vi "UserConsole_Main.vi"(8 "error in (no error)":errorcluster) -> (0 "error out":errorcluster)   [LabVIEW 2013]
doc: "This is Top Level VI for User Console Module. You can communicate with this module using its API. Communication is made based on queue. This module has User Interface so I chase Producer Consumer architecture. In this architecture the User Interface loop is closed using User Event. User Event is sent by Processing (Consumer) loop."
uses:
  General/Controls/#TD_General_CommunicationQueueStates_Enum.ctl
  Private controls/#TD_UserConsole_InnerData_Cluster.ctl
  Private controls/#TD_UserConsole_ModuleStates_Enum.ctl
  Private controls/#TD_UserConsole_ModuleData_Cluster.ctl
  General/Controls/#TD_General_FromWho_Enum.ctl
  General/Controls/#TD_General_UserEventStates_Enum.ctl
  Private controls/#TD_UserConsole_Transactions_Cluster.ctl
  Private controls/#TD_UserConsole_Keys_Cluster.ctl
panel:
  out "CardReader":bool
  in  "Transactions":T1
  in  "blanck_picture":cluster{"Keys":T2, "Screen":string} caption="blank_picture"
  # "[Covers: UI1]"
  # "[Covers: UI2] \n[Covers: UI2A] \n[Covers: UI2B]\n[Covers: UI2C]"
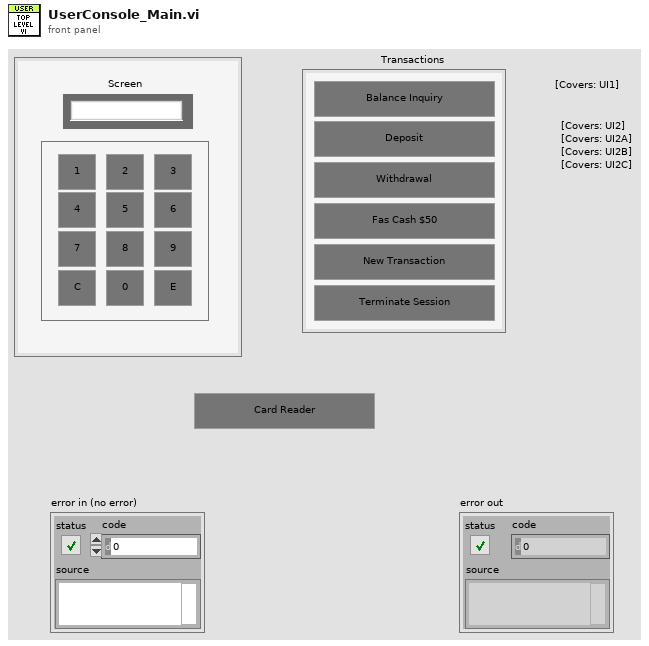
[diagram p1: front panel]
types:
  T1 = typedef "#TD_UserConsole_Transactions_Cluster.ctl" = cluster{"BalanceInquiry":bool, "Deposit":bool, "Withdrawal":bool, "FastCash50":bool, "NewTransaction":bool, "TerminateSession":bool}
  T2 = typedef "#TD_UserConsole_Keys_Cluster.ctl" = cluster{"B1":bool, "B2":bool, "B3":bool, "B4":bool, "B5":bool, "B6":bool, "B7":bool, "B8":bool, "B9":bool, "BC":bool, "B0":bool, "BE":bool}
  T3 = typedef "#TD_General_UserEventStates_Enum.ctl" = enum16{"ERROR_Default", "Create", "GetRef", "Generate", "Release"}
  T4 = typedef "#TD_General_CommunicationQueueStates_Enum.ctl" = enum16{"ERROR_Default", "Obtain", "GetRef", "Enqueue", "EnqueueAtOpp", "GetStatus", "Release"}
  T5 = typedef "#TD_General_FromWho_Enum.ctl" = enum16{"ERROR_Default", "UserConsole", "DisplayConsole", "SensorInterface", "Controller", "Database", "Timing", "ErrorHandling"}
  T6 = typedef "#TD_UserConsole_ModuleStates_Enum.ctl" = enum16{"ERROR_Default", "Init", "Close", "ErrorHandling", "KeyPressed", "TransactionPressed", "CardReaderPressed", "UpdateFP"}
  T7 = typedef "#TD_UserConsole_ModuleData_Cluster.ctl" = cluster{"Action":T6, "Data":variant}
  T8 = typedef "#TD_General_IntermoduleData_Cluster.ctl" = cluster{"Sender":T5, "ModuleData":variant}
  T9 = typedef "#TD_UserConsole_InnerData_Cluster.ctl" = cluster{"Sth":bool, "Screen":string}
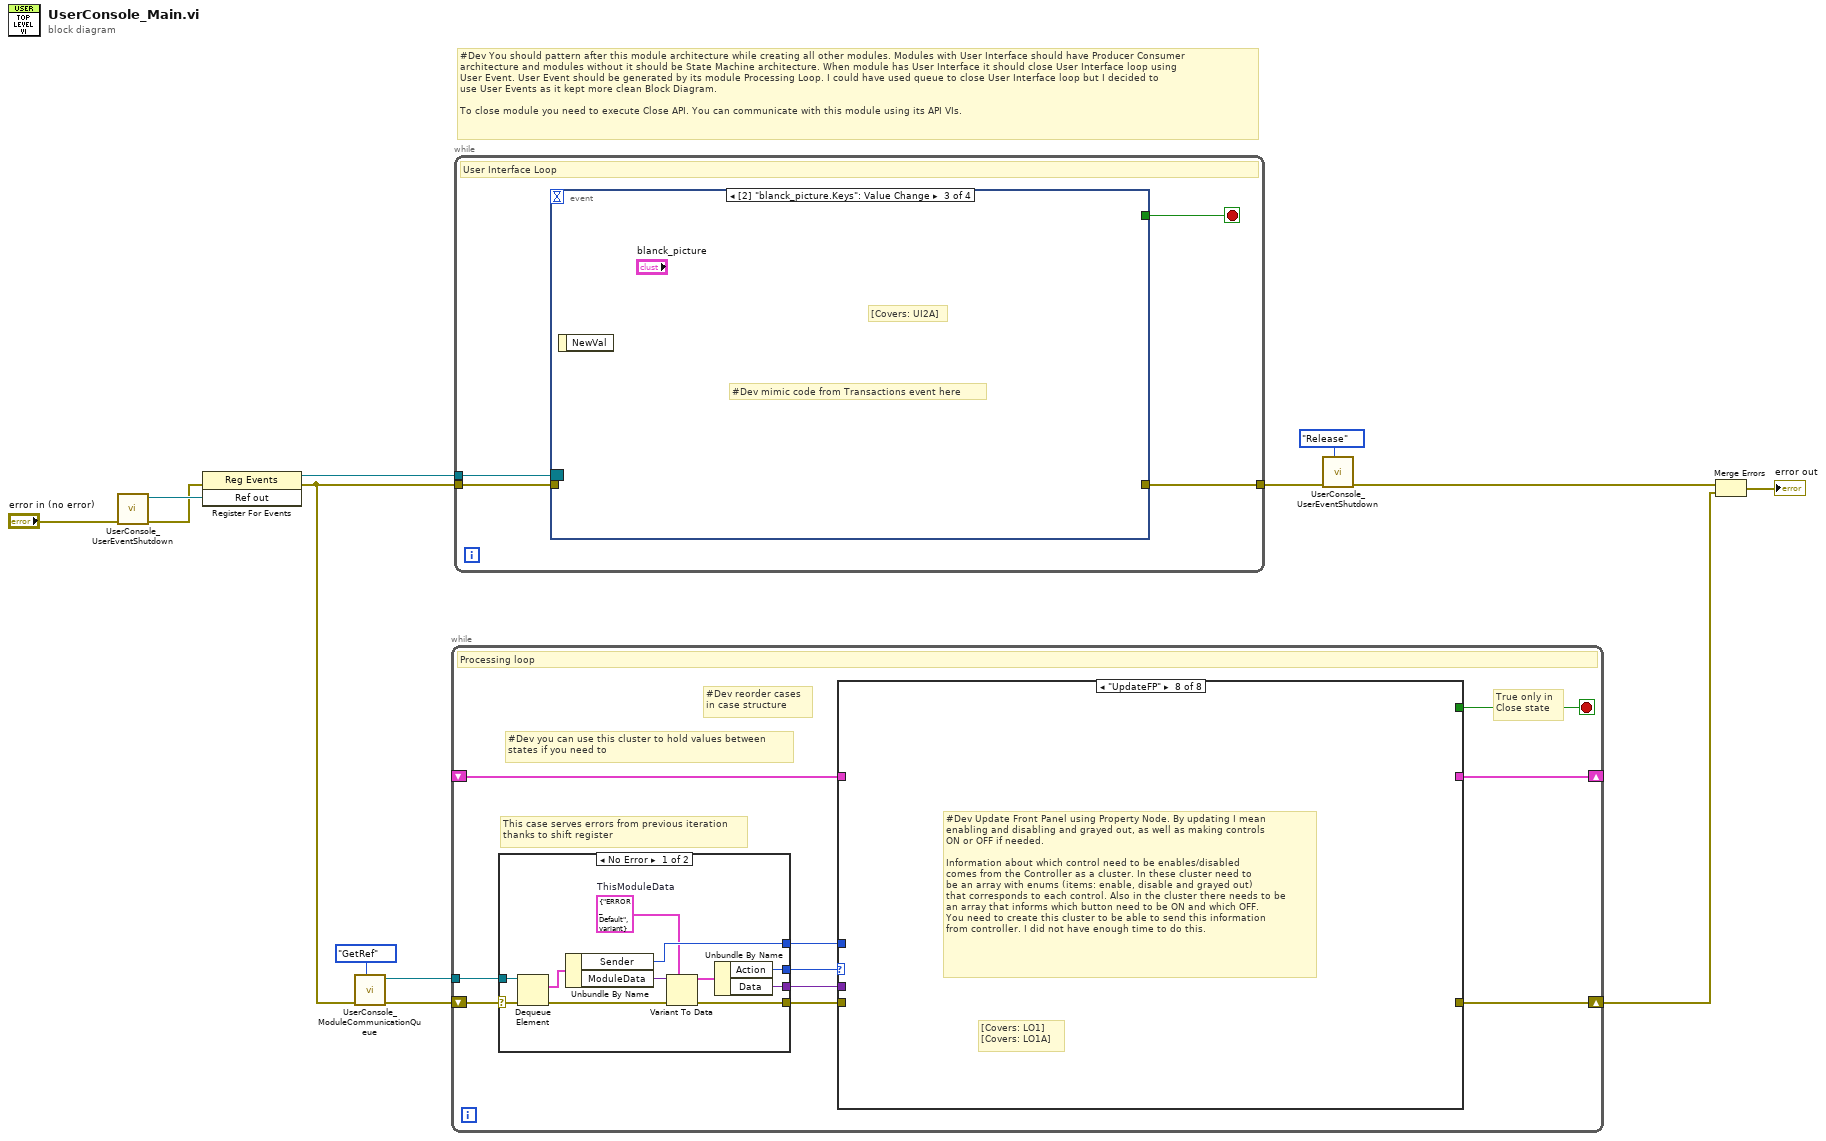
[diagram p0: block diagram]
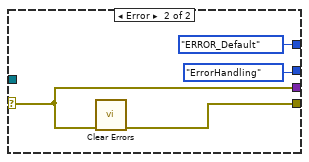
[diagram p2: hidden frame]
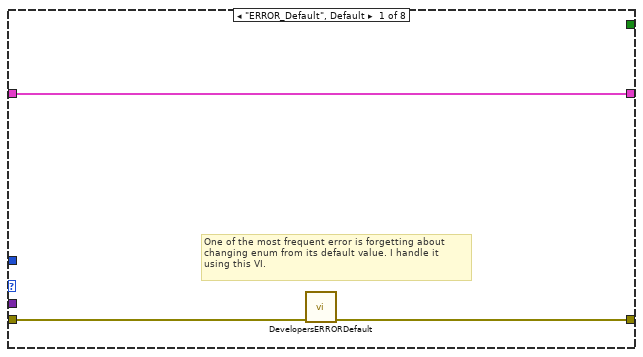
[diagram p3: hidden frame]
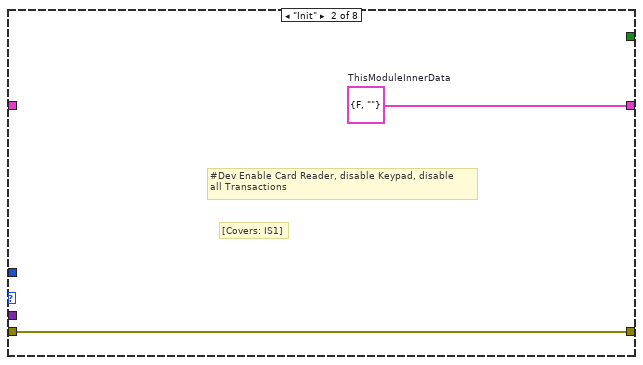
[diagram p4: hidden frame]
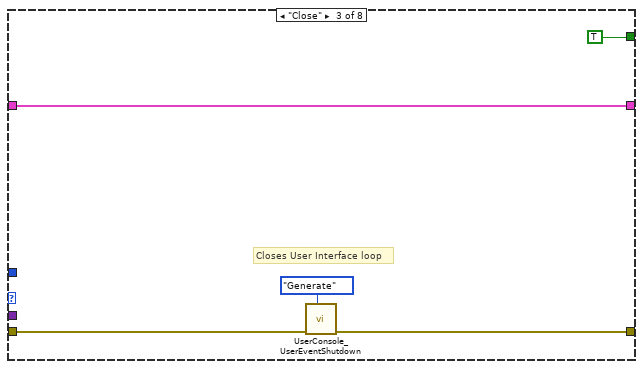
[diagram p5: hidden frame]
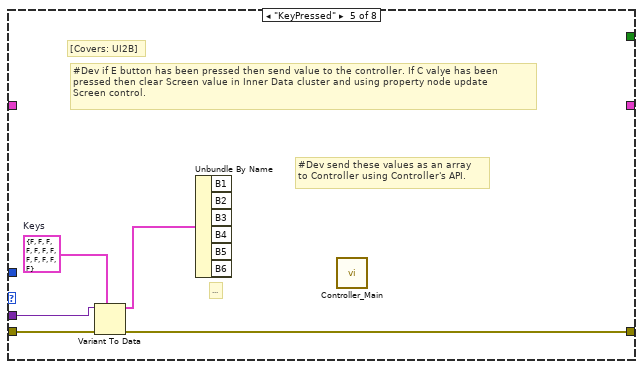
[diagram p7: hidden frame]
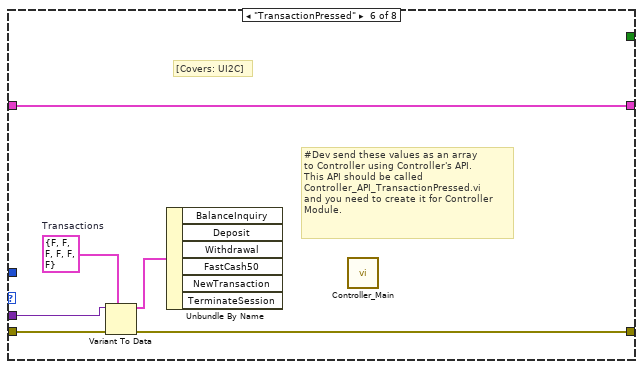
[diagram p8: hidden frame]
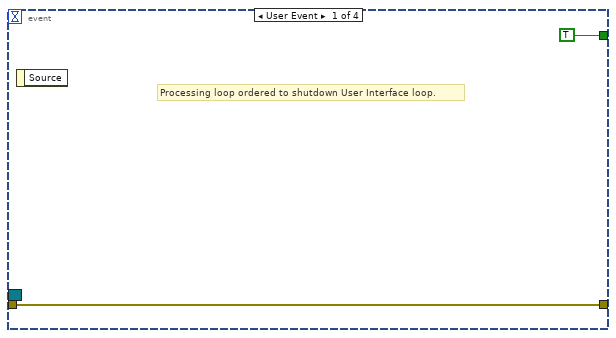
[diagram p10: hidden frame]
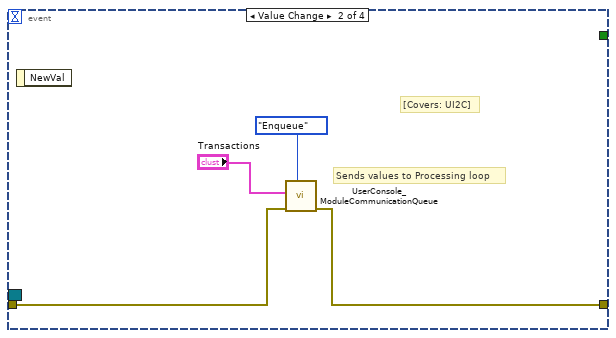
[diagram p11: hidden frame]
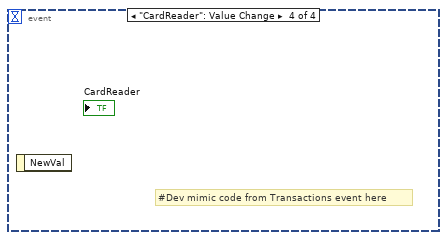
[diagram p12: hidden frame]
diagram:
  # "#Dev You should pattern after this module architecture while creating all other modules. Modules with User Interface should have Producer Consumer \narchitecture and modules without it should be State Machine architecture. When module has User Interface it should close User Interface loop using \nUser Event. User Event should be generated by its module Processing Loop. I could have used queue to close User Interface loop but I decided to \nuse User Events as it kept more clean Block Diagram.\n\nTo close module you need to execute Close API. You can communicate with this module using its API VIs."
  n1 = call "UserConsole_UserEventShutdown.vi"("error in (no error)"="error in (no error)") -> ("error out"=w12:errorcluster, "Ref out"=w13:refnum<user-event>)  [unwired: 9 in]
  n2 = register-events(error in=w12, w13) -> (reference out=w11:refnum<event-registration>, error out=w9:errorcluster)  [unwired: 1 in]
  n3 = call "UserConsole_ModuleCommunicationQueue.vi"("Action"=#TD_General_CommunicationQueueStates_Enum."GetRef", "error in (no error)"=w9) -> ("error out"=w1:errorcluster, "Ref out"=w7:refnum<queue>)  [unwired: 7 in, 1 out]
  n4 = while {
    tunnel: w7 -> [w22]
    shift-right: [w15] -> w3
    shift-left: w1 -> [w23]
    shift-right: [w21] -> _
    shift-left: _ -> [w20]
    stop <- w14 stop-if-true
    # "#Dev reorder cases \nin case structure"
    # "True only in \nClose state"
    # "#Dev you can use this cluster to hold values between \nstates if you need to"
    # "This case serves errors from previous iteration \nthanks to shift register"
    # "Processing loop"
    n5 = case shown="No Error" w23 {
      selector: w23 -> [w34 w38]
      tunnel: w22 -> [w33 _]
      tunnel: [w29 #TD_General_FromWho_Enum."ERROR_Default" ("Sender")] -> w19
      tunnel: [w26 #TD_UserConsole_ModuleStates_Enum."ErrorHandling" ("Action")] -> w18
      tunnel: [w25 w38] -> w17
      tunnel: [w24 w37] -> w16
      frame No Error {
        w28 = T7 {"Action"=enum."ERROR_Default", "Data"=variant}  # ThisModuleData
        n6 = Dequeue Element(queue=w33, error in (no error)=w34) -> (element=w32:T8, error out=w30:errorcluster)  [unwired: 1 in, 2 out]
        n7 = Unbundle By Name(w32) -> ("Sender"=w29:T5, "ModuleData"=w31:variant)
        n8 = Variant To Data(error in=w30, type=w28, Variant=w31) -> (data=w27:T7, error out=w24:errorcluster)
        n9 = Unbundle By Name(w27) -> ("Action"=w26:T6, "Data"=w25:variant)
      }
      frame Error {
        n10 = call <vilib>:"Clear Errors.vi"("error in (no error)"=w38) -> ("error out"=w37:errorcluster)  [unwired: 5 in, 1 out]
      }
    }
    n11 = case shown="\"UpdateFP\"" w18 {
      tunnel: [w41 w43 w47 w50 _ w56 _ _] -> w21
      tunnel: w20 -> [w41 _ w47 w50 _ w56 _ _]
      tunnel: w19 -> [_ _ _ _ _ _ _ _]
      tunnel: w17 -> [_ _ _ _ w54 w58 _ _]
      tunnel: w16 -> [w40 w42 w46 w49 w55 w59 _ _]
      tunnel: [w39 w42 w45 w49 w52 w57 _ _] -> w15
      tunnel: [_ _ TRUE _ _ _ _ _] -> w14
      frame "ERROR_Default", Default {
        # "One of the most frequent error is forgetting about \nchanging enum from its default value. I handle it \nusing this VI."
        n12 = call "DevelopersERRORDefault.vi"("error in (no error)"=w40) -> ("error out"=w39:errorcluster)  [unwired: 10 in]
      }
      frame "Init" {
        w43 = T9 {"Sth"=FALSE, "Screen"=""}  # ThisModuleInnerData
        # "[Covers: IS1]"
        # "#Dev Enable Card Reader, disable Keypad, disable \nall Transactions"
      }
      frame "Close" {
        # "Closes User Interface loop"
        n13 = call "UserConsole_UserEventShutdown.vi"("Action"=#TD_General_UserEventStates_Enum."Generate", "error in (no error)"=w46) -> ("error out"=w45:errorcluster)  [unwired: 8 in, 1 out]
      }
      frame "ErrorHandling" {
        # "#Dev take some actions to handle the error \nand inform central Error Handling Module \nabout this error using Error Handling Module \nAPI"
      }
      frame "KeyPressed" {
        w53 = T2 {"B1"=FALSE, "B2"=FALSE, "B3"=FALSE, "B4"=FALSE, "B5"=FALSE, "B6"=FALSE, "B7"=FALSE, "B8"=FALSE, "B9"=FALSE, "BC"=FALSE, "B0"=FALSE, "BE"=FALSE}  # Keys
        # "#Dev if E button has been pressed then send value to the controller. If C valye has been \npressed then clear Screen value in Inner Data cluster and using property node update \nScreen control."
        # "[Covers: UI2B]"
        # "..."
        # "#Dev send these values as an array \nto Controller using Controller's API."
        n14 = Variant To Data(error in=w55, type=w53, Variant=w54) -> (data=w51:T2, error out=w52:errorcluster)
        n15 = Unbundle By Name(w51) -> ()  [unwired: 6 out]
        n16 = call "Controller_Main.vi"() -> ()  [unwired: 11 in, 1 out]
      }
      frame "TransactionPressed" {
        w61 = T1 {"BalanceInquiry"=FALSE, "Deposit"=FALSE, "Withdrawal"=FALSE, "FastCash50"=FALSE, "NewTransaction"=FALSE, "TerminateSession"=FALSE}  # Transactions
        # "[Covers: UI2C]"
        # "#Dev send these values as an array \nto Controller using Controller's API. \nThis API should be called \nController_API_TransactionPressed.vi \nand you need to create it for Controller \nModule."
        n17 = Variant To Data(error in=w59, type=w61, Variant=w58) -> (data=w60:T1, error out=w57:errorcluster)
        n18 = Unbundle By Name(w60) -> ()  [unwired: 6 out]
        n19 = call "Controller_Main.vi"() -> ()  [unwired: 11 in, 1 out]
      }
      frame "CardReaderPressed" {
        # "[Covers: UI2A]"
        # "#Dev mimic what is done in TransactionPressed state. Pattern after it."
      }
      frame "UpdateFP" {
        # "[Covers: LO1] \n[Covers: LO1A]"
        # "#Dev Update Front Panel using Property Node. By updating I mean \nenabling and disabling and grayed out, as well as making controls \nON or OFF if needed. \n\nInformation about which control need to be enables/disabled \ncomes from the Controller as a cluster. In these cluster need to \nbe an array with enums (items: enable, disable and grayed out) \nthat corresponds to each control. Also in the cluster there needs to be \nan array that informs which button need to be ON and which OFF. \nYou need to create this cluster to be able to send this information \nfrom controller. I did not have enough time to do this."
      }
    }
  }
  n20 = while {
    tunnel: w11 -> [w65]
    tunnel: w9 -> [w63]
    tunnel: [w62] -> w6
    stop <- w64 stop-if-true
    # "User Interface Loop"
    n21 = event shown="[2] \"blanck_picture.Keys\": Value Change" {
      selector: w65 -> [_ _ _ _]
      dyn-events: _ -> [_ _ _ _]
      timeout: _ -> [_ _ _ _]
      tunnel: [TRUE _ _ _] -> w64
      tunnel: w63 -> [w66 w71 _ _]
      tunnel: [w66 w68 _ _] -> w62
      event User Event {
        # "Processing loop ordered to shutdown User Interface loop."
        n22 = event-data() -> ()  [unwired: 1 in, 1 out]
      }
      event Value Change {
        # "[Covers: UI2C]"
        # "Sends values to Processing loop"
        n23 = event-data() -> ()  [unwired: 1 in, 1 out]
        n24 = call "UserConsole_ModuleCommunicationQueue.vi"("Action"=#TD_General_CommunicationQueueStates_Enum."Enqueue", "error in (no error)"=w71, "ModuleData"="Transactions") -> ("error out"=w68:errorcluster)  [unwired: 6 in, 2 out]
      }
      event Value Change {
        # "[Covers: UI2A]"
        # "#Dev mimic code from Transactions event here"
        n25 = event-data() -> ()  [unwired: 1 in, 1 out]
      }
      event "CardReader": Value Change {
        # "#Dev mimic code from Transactions event here"
        n26 = event-data() -> ()  [unwired: 1 in, 1 out]
      }
    }
  }
  n27 = call "UserConsole_UserEventShutdown.vi"("Action"=#TD_General_UserEventStates_Enum."Release", "error in (no error)"=w6) -> ("error out"=w4:errorcluster)  [unwired: 8 in, 1 out]
  n28 = Merge Errors(w4, w3) -> (→"error out":errorcluster)
